vi "Write to.vi"(11 "变体":variant) -> ()   [LabVIEW 2018]
uses:
  <vilib>/Utility/xml.llb/Write to XML File(string).vi
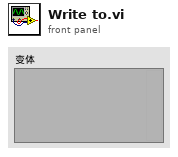
[diagram p1: front panel]
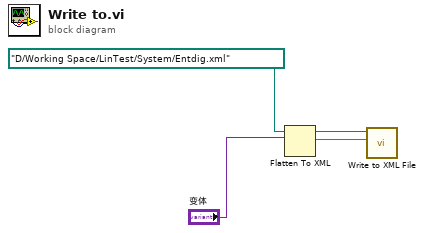
[diagram p0: block diagram]
diagram:
  n1 = Flatten To XML(anything="变体") -> (xml string=w3:string)
  n2 = call-poly <vilib>:"Write to XML File.vi"("XML Input"=w3, "XML File Path"=path "D:/Working Space/LinTest/System/Entdig.xml") -> ()  [unwired: 7 in, 3 out]
